vi "Graph_AO.vi"(8 "error in":errorcluster, 11 "Square Wave":T1) -> (0 "error out":errorcluster)   [LabVIEW 2019]
uses:
  Set_AO_Wave-config.ctl
panel:
  in  "Exit":bool
  out "wfm":waveform(dbl)(graph)
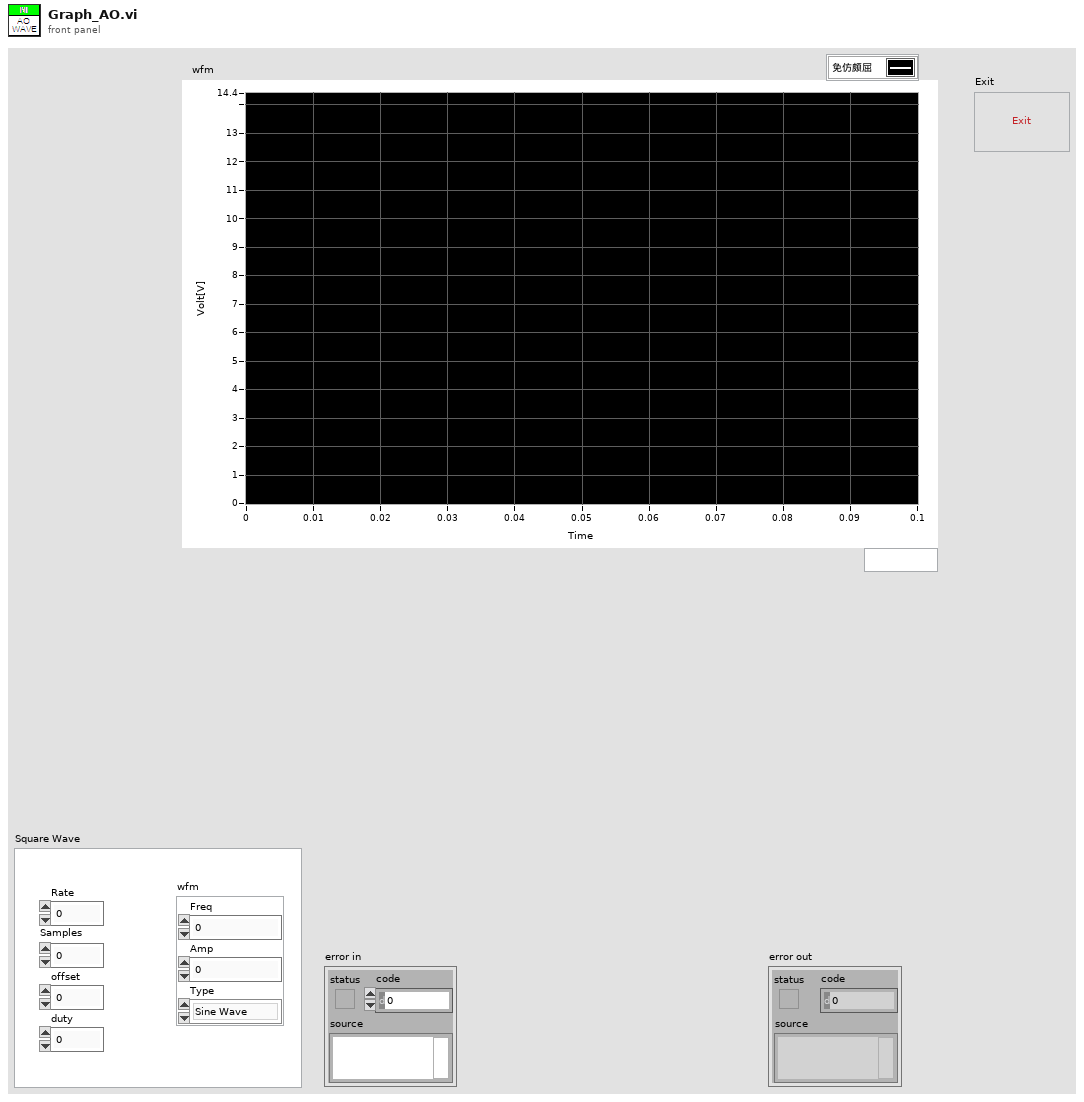
[diagram p1: front panel]
types:
  T1 = typedef "Set_AO_Wave-config.ctl" = cluster{"offset":dbl, "Samples":i32, "duty":dbl, "Rate":dbl, "wfm":cluster{"Freq":dbl, "Amp":dbl, "Type":enum16{"Sine Wave", "Triangle Wave", "Square Wave", "Sawtooth Wave"}}}
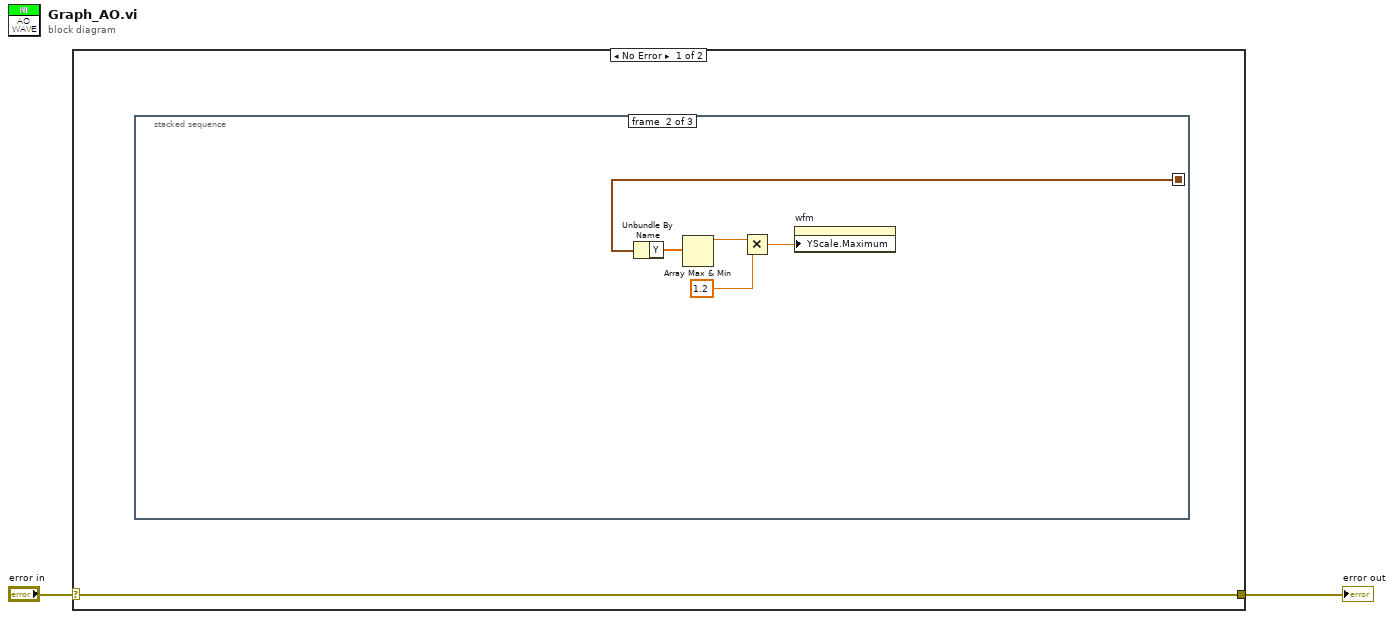
[diagram p0: block diagram]
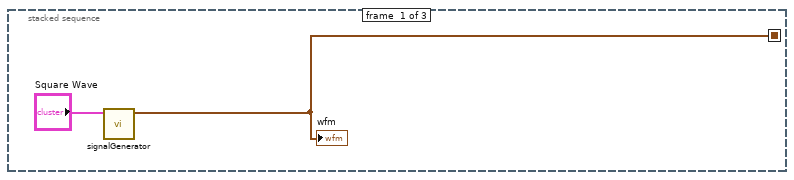
[diagram p2: hidden frame]
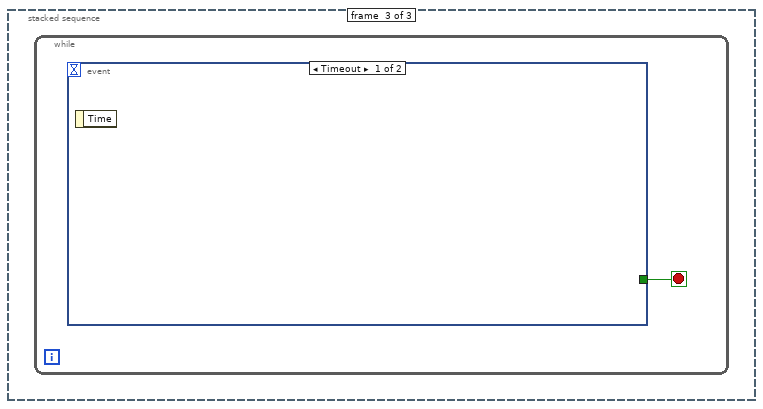
[diagram p3: hidden frame]
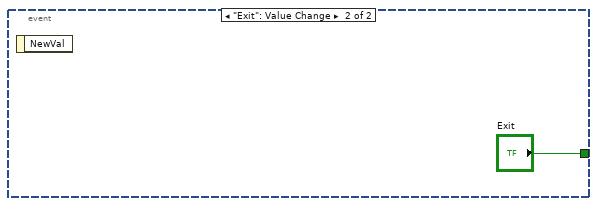
[diagram p4: hidden frame]
diagram:
  n1 = case shown="No Error" "error in" {
    selector: "error in" -> [w3 w13]
    tunnel: [w3 w13] -> w1
    frame No Error {
      n2 = stacked-sequence {
        seq-local: [w4 _ _] -> [_ w7 _]
        frame #0 {
          n3 = call "signalGenerator.vi"("Square Wave"="Square Wave") -> ("signal out_display"=w4:waveform(dbl))  [unwired: 9 in, 1 out]
          "wfm" <- w4
        }
        frame #1 {
          n4 = Unbundle By Name(w7) -> ("Y"=w6:dbl[])
          n5 = Array Max & Min(array=w6) -> (max value=w10:dbl)  [unwired: 3 out]
          n6 = Multiply(x=w10, y=1.2) -> (x*y=w9:dbl)
          n7 = property on="wfm" class="WFGraph (strict)"("YScale.Maximum"=w9) -> ()  [unwired: 2 in, 2 out]
        }
        frame #2 {
          n8 = while {
            stop <- w11 stop-if-true
            n9 = event shown="[0] Timeout" {
              selector: _ -> [_ _]
              dyn-events: _ -> [_ _]
              timeout: _ -> [_ _]
              tunnel: [_ "Exit"] -> w11
              event Timeout {
                n10 = event-data() -> ()  [unwired: 1 in, 1 out]
              }
              event "Exit": Value Change {
                n11 = event-data() -> ()  [unwired: 1 in, 1 out]
              }
            }
          }
        }
      }
    }
    frame Error {
    }
  }
  "error out" <- w1
